vi "AssertStringContainsString.vi"(5 "Needle":string, 7 "Message (\"\")":string, 8 "error in (no error)":errorcluster, 10 "Haystack":string) -> (0 "error out":errorcluster, 2 "Result":bool)   [LabVIEW 2019, in "Assertion.lvlib"]
doc: "Asserts that <B>haystack</B> contains <B>needle</B>. Does nothing if an error occurred before this node runs. Returns an error if the assertion failed. Optionally adds a message to the error message if the assertion failed."
uses:
  Assertion.lvlib
  Constraint/StringContains/StringContains.lvclass
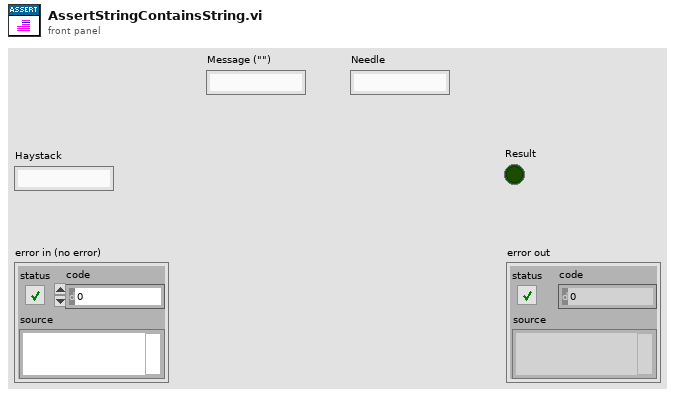
[diagram p1: front panel]
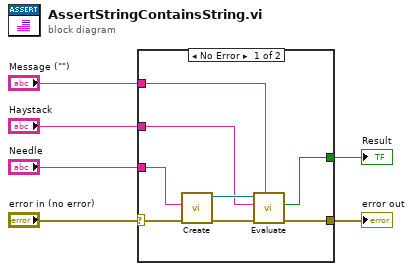
[diagram p0: block diagram]
diagram:
  n1 = case shown="No Error" "error in (no error)" {
    selector: "error in (no error)" -> [w8 w15]
    tunnel: "Haystack" -> [w12 _]
    tunnel: [w11 w15] -> w5
    tunnel: [w10 _] -> w4
    tunnel: "Message (\"\")" -> [w9 _]
    tunnel: "Needle" -> [w7 _]
    frame No Error {
      n2 = call "Create.vi"("error in (no error)"=w8, "Needle"=w7) -> ("error out"=w13:errorcluster, "StringContains"=w14:refnum<class "StringContains.lvclass">)  [unwired: 8 in]
      n3 = call-dynamic "Evaluate.vi"("Message (\"\")"=w9, "error in (no error)"=w13, "Actual"=w12, "Constraint in"=w14) -> ("error out"=w11:errorcluster, "Result"=w10:bool)  [unwired: 5 in, 1 out]
    }
    frame Error {
    }
  }
  "error out" <- w5
  "Result" <- w4
